vi "readLogILCCommunication.vi"(8 "error in (no error)":errorcluster, 10 "Parser":refnum<class "U8ArrayParserAutoIndexing.lvclass">, 11 "M1M3SAL in":refnum<class "M1M3SAL.lvclass">) -> (0 "error out":errorcluster, 2 "EventILCCommunication":variant, 3 "M1M3SAL out":refnum<class "M1M3SAL.lvclass">)   [LabVIEW 2016, in "M1M3SupportCommunicator.lvlib" / "M1M3SAL.lvclass"]
uses:
  M1M3SAL.lvclass
  Common_RT_Utilities/U8ArrayParserAutoIndexing/U8ArrayParserAutoIndexing.lvclass
  DataTypes/Topics/EventILCCommunication.ctl
  DataTypes/Topics/Parts/Timestamp.ctl
  DataTypes/Topics/M1M3SupportTopics.lvlib
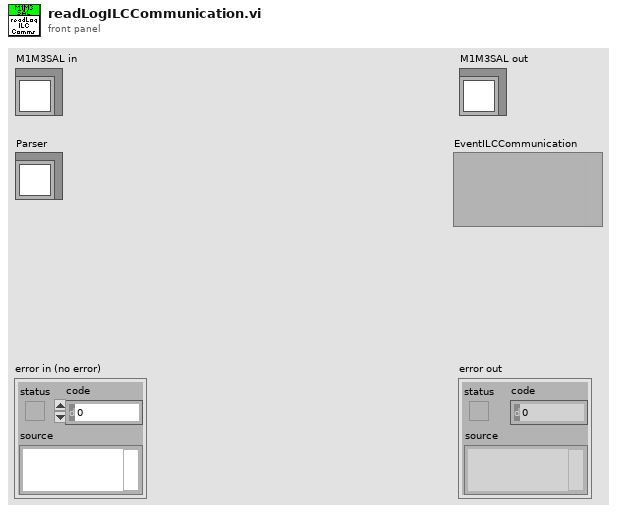
[diagram p1: front panel]
types:
  T1 = typedef "M1M3SupportTopics.lvlib/EventILCCommunication.ctl" = cluster{"Timestamp":T2, "ActuatorId":i32, "CommunicationOK":bool}
  T2 = typedef "M1M3SupportTopics.lvlib/Timestamp.ctl" = dbl
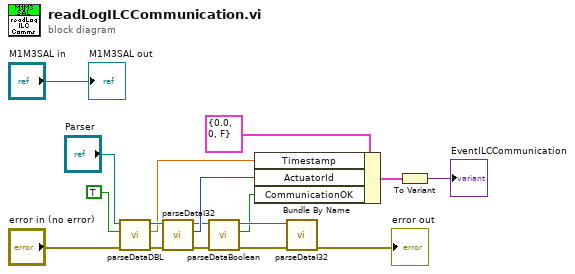
[diagram p0: block diagram]
diagram:
  n1 = call "parseDataDBL.vi"("error in (no error)"="error in (no error)", "OverrideSwapBytes"=TRUE, "U8ArrayParserAutoIndexing in"="Parser") -> ("error out"=w9:errorcluster, "Data"=w7:dbl, "U8ArrayParserAutoIndexing out"=w8:refnum<class "U8ArrayParserAutoIndexing.lvclass">)  [unwired: 6 in]
  n2 = call "parseDataI32.vi"("error in (no error)"=w9, "U8ArrayParserAutoIndexing in"=w8) -> ("error out"=w4:errorcluster, "Data"=w14:i32, "U8ArrayParserAutoIndexing out"=w5:refnum<class "U8ArrayParserAutoIndexing.lvclass">)  [unwired: 7 in]
  n3 = call "parseDataBoolean.vi"("error in (no error)"=w4, "U8ArrayParserAutoIndexing in"=w5) -> ("error out"=w2:errorcluster, "Data"=w1:bool, "U8ArrayParserAutoIndexing out"=w3:refnum<class "U8ArrayParserAutoIndexing.lvclass">)  [unwired: 7 in]
  n4 = Bundle By Name(cluster=T1 {"Timestamp"=0.0, "ActuatorId"=0, "CommunicationOK"=FALSE} ("EventILCCommunication"), "Timestamp"=w7, "ActuatorId"=w14, "CommunicationOK"=w1) -> (w16:T1)
  n5 = call "parseDataI32.vi"("error in (no error)"=w2, "U8ArrayParserAutoIndexing in"=w3) -> ("error out"=→"error out":errorcluster)  [unwired: 7 in, 2 out]
  n6 = To Variant(anything=w16) -> (Variant=→"EventILCCommunication":variant)
  "M1M3SAL out" <- "M1M3SAL in"
